vi "Configure LAN Trigger Input Line.vi"(8 "error in (no error)":errorcluster, 9 "Detected Edge":u16(ring) items=["Falling", "Rising", "Either"], 10 "LAN Event Number (1)":u32=1 min=1 max=8 step=1, 11 "VISA resource name":refnum<visa-resource-name>) -> (0 "error out":errorcluster, 3 "VISA resource name out":refnum<visa-resource-name>)   [LabVIEW 2021, in "Keithley DMM7510.lvlib"]
doc: "This VI sets the logic on which the trigger event detector and the output trigger generator operate on the given trigger line."
uses:
  Keithley DMM7510.lvlib
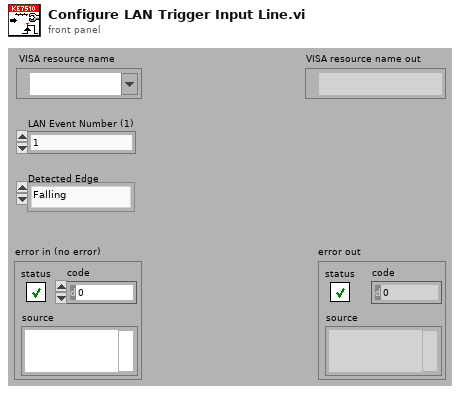
[diagram p1: front panel]
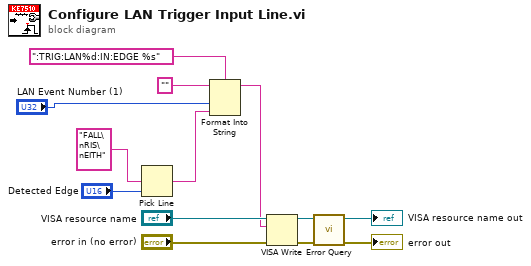
[diagram p0: block diagram]
diagram:
  n1 = Pick Line(multi-line string="FALL\nRIS\nEITH", line index="Detected Edge") -> (output string=w2:string)  [unwired: 1 in]
  n2 = Format Into String(format string=":TRIG:LAN%d:IN:EDGE %s", initial string="", "LAN Event Number (1)", w2) -> (resulting string=w5:string)  [unwired: 1 in, 1 out]
  n3 = VISA Write(VISA resource name="VISA resource name", write buffer=w5, error in (no error)="error in (no error)") -> (VISA resource name out=w9:refnum<visa-resource-name>, error out=w8:errorcluster)  [unwired: 1 out]
  n4 = call "Error Query.vi"("error in (no error)"=w8, "VISA resource name"=w9) -> ("error out"=→"error out":errorcluster, "VISA resource name out"=→"VISA resource name out":refnum<visa-resource-name>)  [unwired: 8 out]
